vi "Project simulated.vi"() -> ()   [LabVIEW 2023]
uses:
  <vilib>/addons/control/pid/pid.llb/PID (DBL).vi
  <vilib>/addons/control/pid/NI_PID_pid.lvlib
panel:
  out "u":dbl format="%_2g V"
  out "Tout":dbl format="%_4f °C"
  in  "Ts":dbl
  out "Waveform Chart":dbl(graph)
  in  "Initial Value":dbl
  in  "Set Point":dbl
  in  "Stop Button":bool
  in  "PID Controller":cluster{"Kp":dbl, "Ti":dbl, "Td":dbl}
  # "Temperature"
  # "Time"
  # "PID Control"
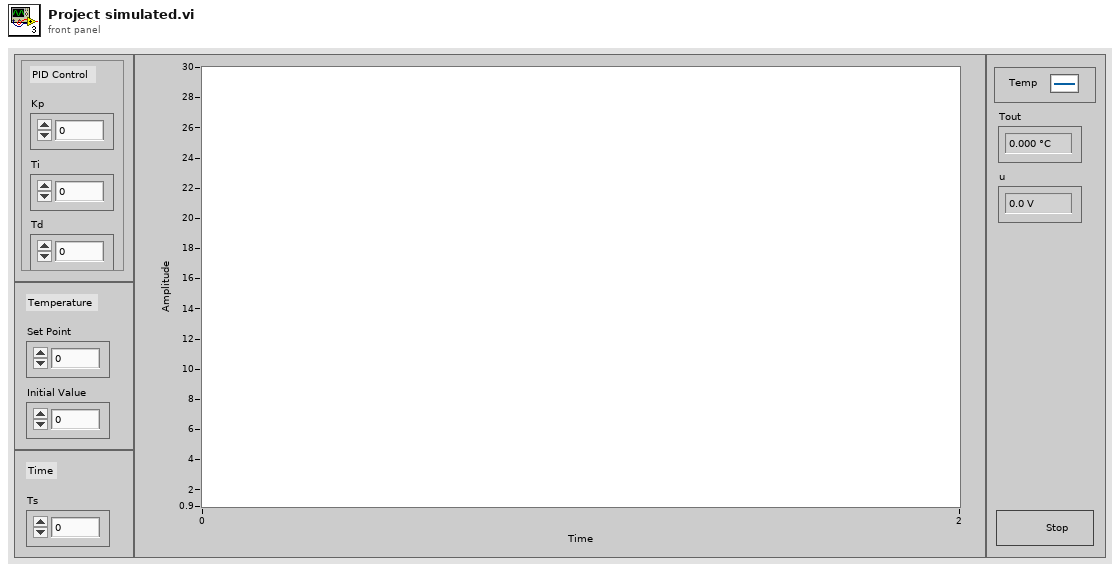
[diagram p1: front panel]
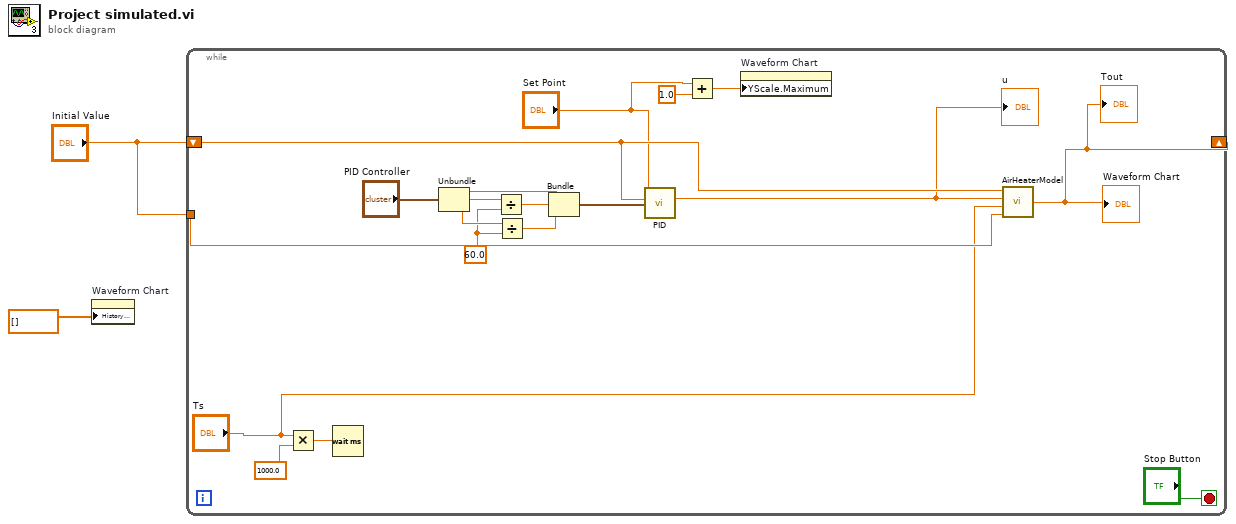
[diagram p0: block diagram]
diagram:
  n1 = property on="Waveform Chart" class="WFChart (strict)"("History Data"=dbl[] []) -> ()  [unwired: 2 in, 2 out]
  n2 = while {
    shift-right: [w4] -> _
    shift-left: "Initial Value" -> [w10]
    tunnel: "Initial Value" -> [w9]
    stop <- "Stop Button" stop-if-true
    w17 = 60.0 ("y")
    n3 = Multiply(x="Ts", y=1000.0) -> (x*y=w11:dbl)
    n4 = Wait (ms)(milliseconds to wait=w11) -> ()  [unwired: 1 out]
    n5 = Unbundle("PID Controller") -> ("Kp"=w15:dbl, "Ti"=w19:dbl, "Td"=w18:dbl)
    n6 = Divide(x=w19, y=w17) -> (x/y=w16:dbl)
    n7 = Divide(x=w18, y=w17) -> (x/y=w14:dbl)
    n8 = Bundle("Kp"=w15, w16, w14) -> (w13:cluster{"Kp":dbl, dbl, dbl})  [unwired: 1 in]
    n9 = call-poly <vilib>:"PID.vi"("PID gains"=w13, "process variable"=w10, "setpoint"="Set Point") -> ("output"=w3:dbl)  [unwired: 7 in, 1 out]
    "u" <- w3
    n10 = Add(x="Set Point", y=1.0) -> (x+y=w6:dbl)
    n11 = property on="Waveform Chart" class="WFChart (strict)"("YScale.Maximum"=w6) -> ()  [unwired: 2 in, 2 out]
    n12 = call "AirHeaterModel.vi"("Tenv"=w9, "Ts"="Ts", "u"=w3, "Tout"=w10) -> ("Tout"=w4:dbl)
    "Waveform Chart" <- w4
    "Tout" <- w4
  }
